vi "sub_save.vi"   [LabVIEW 2016]
uses:
  ctl/UI_cmd-ctl.ctl
  Global.vi
types:
  T1 = typedef "UI_cmd-ctl.ctl" = enum16{"default", "create", "read"}
  T2 = typedef "data.ctl" = cluster{"Bonding force":dbl, "Bonding time":dbl, "Bonding index":dbl, "Pickup force":dbl, "Pickup time":dbl, "Pickup index":dbl, "Detach force":dbl, "Detach time":dbl, "Detach index":dbl, "Heater temp rt":dbl, "Vacuum rt":dbl, "IR raw data":i16[][], "IR temp data":dbl[][], "vacuum raw wf":waveform(dbl), "vacuum kpa wf":waveform(dbl), "strain raw wf":waveform(dbl)[], "Force rt":dbl, "Vacuum T":dbl, "Heater temp T":dbl, "Balance xy arrays":cluster{dbl, dbl}[], "Balance xy":cluster{dbl, dbl}[], "Bonding wf index":dbl, "Pickup wf index":dbl, "Bonding rising index":dbl, "Bonding falling index":dbl, "Pickup rising index":dbl, "Pickup falling index":dbl}
  T3 = typedef "UI_ctl.ctl" = cluster{"Heater temp":refnum<vi>, "Heater chart":refnum<vi>, "vacuum (kpa)":refnum<vi>, "Balance xy graph":refnum<vi>, "Strain chart w cal":refnum<vi>, "Pickup force":refnum<vi>, "Pickup time":refnum<vi>, "Force chart":refnum<vi>, "Force graph T":refnum<vi>, "vacuum chart":refnum<vi>, "vacuum rt":refnum<vi>, "Strain raw graph":refnum<vi>, "Strain raw chart":refnum<vi>, "Bonding time":refnum<vi>, "Bonding force":refnum<vi>, "Balance":refnum<vi>, "Filtered force graph":refnum<vi>, "ROI intensity":refnum<vi>, "Heater_rt":refnum<vi>, "Detach force":refnum<vi>, "Force rt":refnum<vi>, "Mixed signal":refnum<vi>}
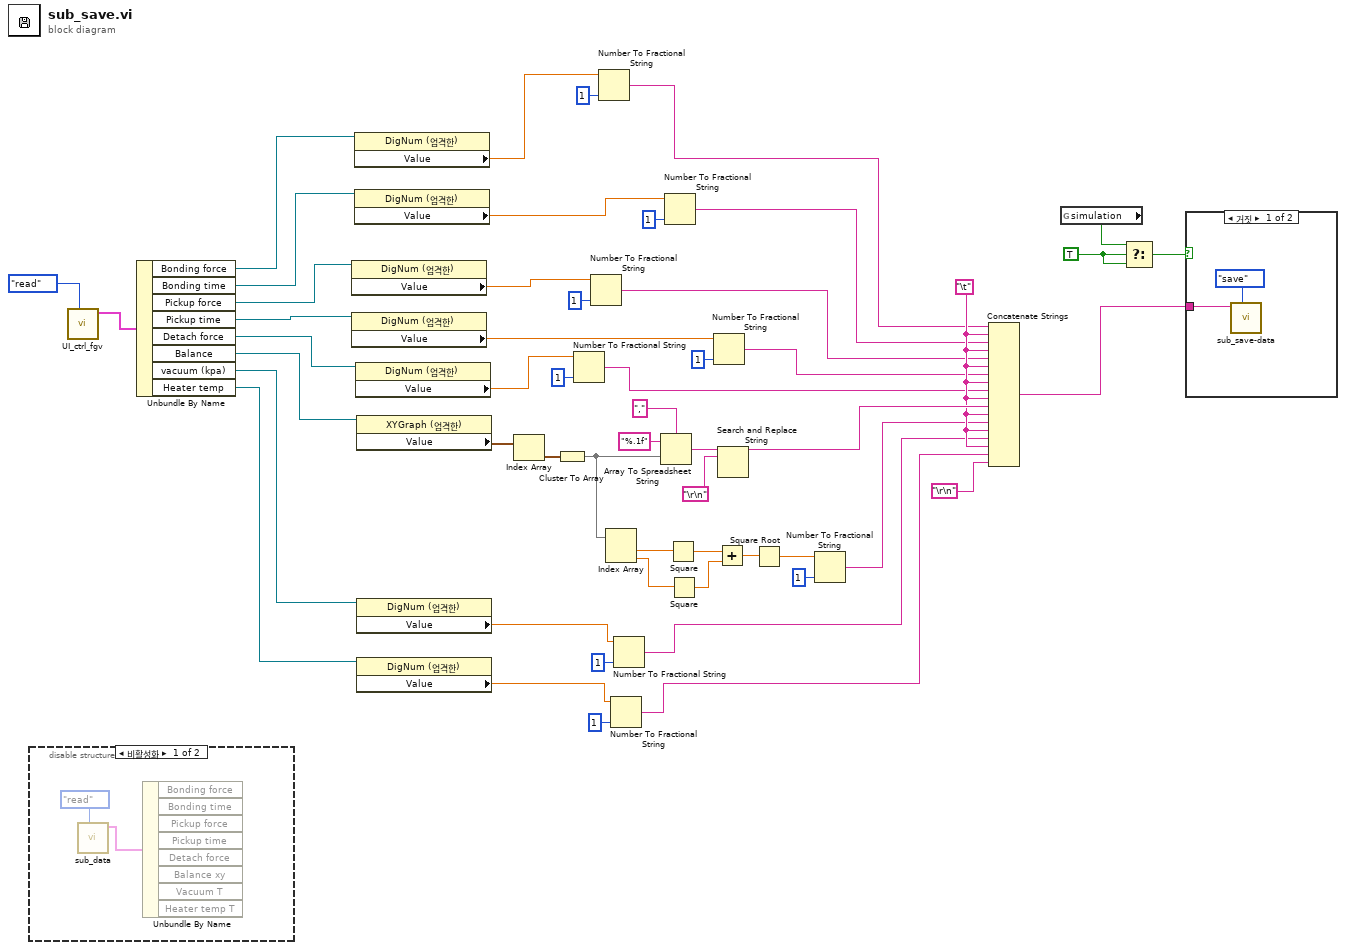
[diagram p0: block diagram]
diagram:
  w33 = TRUE
  w25 = "\t"
  n1 = disable-structure shown="비활성화" {
    frame Disabled {
      n2 = call "sub_data.vi"("cmd"=enum16{"ini", "write", "read"}."read") -> ("data out"=w54:T2)  [unwired: 9 in, 1 out]
      n3 = Unbundle By Name(w54) -> ()  [unwired: 8 out]
    }
    frame Enabled {
    }
  }
  n4 = call "UI_ctrl_fgv.vi"("cmd"=UI_cmd-ctl."read") -> ("UI cluster out"=w46:T3)  [unwired: 10 in]
  n5 = Unbundle By Name(w46) -> ("Bonding force"=w48:refnum<vi>, "Bonding time"=w41:refnum<vi>, "Pickup force"=w39:refnum<vi>, "Pickup time"=w38:refnum<vi>, "Detach force"=w36:refnum<vi>, "Balance"=w40:refnum<vi>, "vacuum (kpa)"=w45:refnum<vi>, "Heater temp"=w53:refnum<vi>)
  n6 = property class="DigNum (엄격한)"(reference=w39) -> ("Value"=w17:dbl)  [unwired: 1 in, 2 out]
  n7 = property class="DigNum (엄격한)"(reference=w38) -> ("Value"=w5:dbl)  [unwired: 1 in, 2 out]
  n8 = property class="DigNum (엄격한)"(reference=w48) -> ("Value"=w20:dbl)  [unwired: 1 in, 2 out]
  n9 = property class="DigNum (엄격한)"(reference=w41) -> ("Value"=w2:dbl)  [unwired: 1 in, 2 out]
  n10 = property class="DigNum (엄격한)"(reference=w36) -> ("Value"=w14:dbl)  [unwired: 1 in, 2 out]
  n11 = property class="XYGraph (엄격한)"(reference=w40) -> ("Value"=w44:cluster{"X":dbl, "Y":dbl}[])  [unwired: 1 in, 2 out]
  n12 = property class="DigNum (엄격한)"(reference=w45) -> ("Value"=w11:dbl)  [unwired: 1 in, 2 out]
  n13 = property class="DigNum (엄격한)"(reference=w53) -> ("Value"=w8:dbl)  [unwired: 1 in, 2 out]
  n14 = Index Array(array=w44) -> (element=w43:cluster{"X":dbl, "Y":dbl})  [unwired: 1 in]
  n15 = Cluster To Array(cluster=w43) -> (array=w31:dbl[])
  n16 = Number To Fractional String(number=w14, precision (6)=i16 1 ("정밀도(6)")) -> (F-format string=w13:string)  [unwired: 2 in]
  n17 = Number To Fractional String(number=w17, precision (6)=i16 1 ("정밀도(6)")) -> (F-format string=w16:string)  [unwired: 2 in]
  n18 = Number To Fractional String(number=w20, precision (6)=i16 1 ("정밀도(6)")) -> (F-format string=w19:string)  [unwired: 2 in]
  n19 = Index Array(array=w31) -> (element #1=w30:dbl, element #2=w29:dbl)  [unwired: 2 in]
  n20 = Number To Fractional String(number=w8, precision (6)=i16 1 ("정밀도(6)")) -> (F-format string=w7:string)  [unwired: 2 in]
  n21 = Number To Fractional String(number=w11, precision (6)=i16 1 ("정밀도(6)")) -> (F-format string=w10:string)  [unwired: 2 in]
  n22 = Array To Spreadsheet String(delimiter (Tab)="," ("구분 문자(탭)"), array=w31, 3:"%.1f" ("포맷 문자열")) -> (spreadsheet string=w50:string)
  n23 = Number To Fractional String(number=w2, precision (6)=i16 1 ("정밀도(6)")) -> (F-format string=w1:string)  [unwired: 2 in]
  n24 = Square(x=w30) -> (x^2=w28:dbl)
  n25 = Square(x=w29) -> (x^2=w27:dbl)
  n26 = Number To Fractional String(number=w5, precision (6)=i16 1 ("정밀도(6)")) -> (F-format string=w4:string)  [unwired: 2 in]
  n27 = Add(x=w28, y=w27) -> (x+y=w26:dbl)
  n28 = Search and Replace String(input string=w50, search string="\r\n") -> (result string=w37:string)  [unwired: 6 in, 3 out]
  n29 = Square Root(x=w26) -> (sqrt(x)=w24:dbl)
  n30 = Number To Fractional String(number=w24, precision (6)=i16 1 ("정밀도(6)")) -> (F-format string=w23:string)  [unwired: 2 in]
  n31 = Concatenate Strings(w19, w25, w1, w25, w16, w25, w4, w25, w13, w25, w37, w25, w23, w25, w10, w25, w7, "\r\n") -> (w51:string)
  n32 = global read "Global.vi" "simulation"() -> (w35:bool)
  n33 = Select(t=w35, s=w33, f=w33) -> (s? t:f=w34:bool)
  n34 = case shown="거짓" w34 {
    tunnel: w51 -> [w57 _]
    frame False {
      n35 = call "sub_save-data.vi"("cmd"=enum16{"create", "save"}."save", "data"=w57) -> ()  [unwired: 9 in, 1 out]
    }
    frame True {
    }
  }
